vi "setParameter.vi"(8 "error in (no error)":errorcluster, 9 "DeviceParm":u8[](array[numeric]), 10 "Device":i32, 11 "SEDSpectrometer in":refnum<class "FiberSpectrograph.lvclass">) -> (0 "error out":errorcluster, 1 "DeviceParm":u8[](array[numeric]), 2 "Output Value":i32, 3 "SEDSpectrometer out":refnum<class "FiberSpectrograph.lvclass">)   [LabVIEW 2016, in "FiberSpectrograph.lvclass"]
uses:
  FiberSpectrograph.lvclass
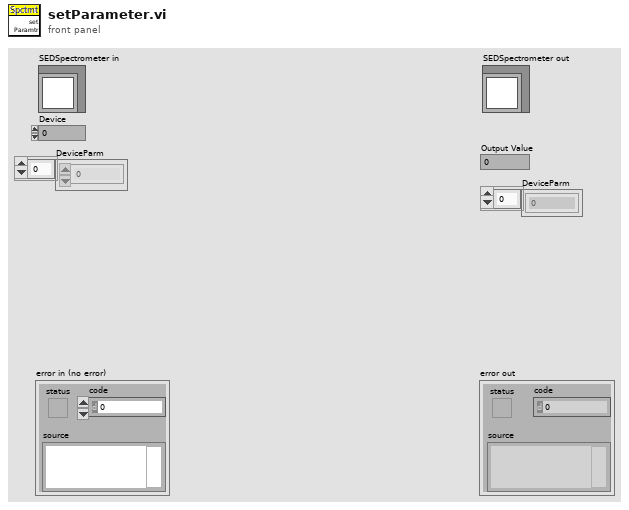
[diagram p1: front panel]
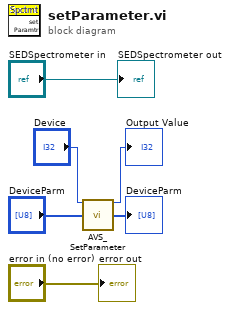
[diagram p0: block diagram]
diagram:
  n1 = call "AVS_SetParameter.vi"("a_hDevice"="Device", "a_pDeviceParm"="DeviceParm") -> ("Output Value"=→"Output Value":i32, "a_pDeviceParm"=→"DeviceParm":u8[])  [unwired: 12 in]
  "error out" <- "error in (no error)"
  "SEDSpectrometer out" <- "SEDSpectrometer in"
